vi "openShutter.vi"(11 "VISA Refnum in":refnum<visa-resource-name>) -> (0 "error out":errorcluster, 3 "VISA Refnum out":refnum<visa-resource-name>)   [LabVIEW 2021]
doc: "Newport Motion Controler\nOpen Shutter communication port\n\nAndré Romero - 2020\nandretec@ifsc.usp.br"
uses:
  <vilib>/Instr/_visa.llb/VISA Configure Serial Port (Instr).vi
  Global Shutter.vi
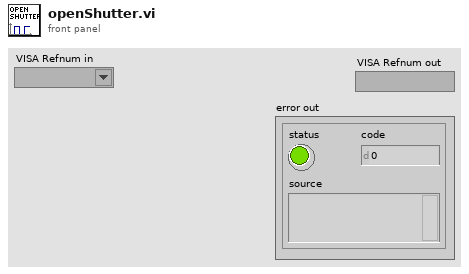
[diagram p1: front panel]
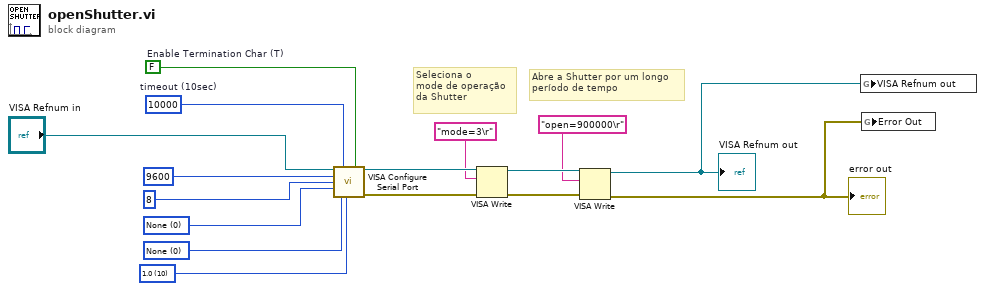
[diagram p0: block diagram]
diagram:
  w8 = u16 0 items=["None", "Odd", "Even", "Mark", "Space"] ("parity")
  w5 = u16 10 items=["1.0"=10, "1.5"=15, "2.0"=20] ("stop bits")
  w4 = u16 0 items=["None"=0, "XON/XOFF"=1, "RTS/CTS"=2, "DTR/DSR"=4] ("flow control")
  w6 = FALSE  # Enable Termination Char (T)
  w7 = u32 10000  # timeout (10sec)
  # "Abre a Shutter por um longo\nperíodo de tempo"
  # "Seleciona o \nmode de operação\nda Shutter"
  n1 = call-poly "VISA Configure Serial Port"("VISA resource name"="VISA Refnum in", "timeout (10sec)"=w7, "Enable Termination\nChar (T)"=w6, "baud rate (9600)"=u32 9600 ("baud rate"), "data bits (8)"=u16 8 ("data bits"), "parity (0:none)"=w8, "stop bits (10: 1 bit)"=w5, "flow control (0:none)"=w4) -> ("VISA resource name out"=w12:refnum<visa-resource-name>, "error out"=w13:errorcluster)  [unwired: 6 in]
  n2 = VISA Write(VISA resource name=w12, write buffer="mode=3\r", error in (no error)=w13) -> (VISA resource name out=w15:refnum<visa-resource-name>, error out=w16:errorcluster)  [unwired: 1 out]
  n3 = VISA Write(VISA resource name=w15, write buffer="open=900000\r", error in (no error)=w16) -> (VISA resource name out=w2:refnum<visa-resource-name>, error out=w1:errorcluster)  [unwired: 1 out]
  "error out" <- w1
  "VISA Refnum out" <- w2
  n4 = global write "Global Shutter.vi" "VISA Refnum out"(w2) -> ()
  n5 = global write "Global Shutter.vi" "Error Out"(w1) -> ()
